vi "Test_Create.vi"(8 "error in (no error)":errorcluster, 11 "TestCase in":refnum<class "StringList_Delegations.lvclass">) -> (0 "error out":errorcluster, 3 "TestCase out":refnum<class "StringList_Delegations.lvclass">)   [LabVIEW 2009, in "StringList_Delegations.lvclass"]
uses:
  StringList_Delegations.lvclass
  Test Doubles/ListImp_RefSpy/ListImp_RefSpy.lvclass
  source/Lists.Interfaces/StringList/StringList.lvclass
  UnitTestComparisons/UnitTestComparisons.lvlib
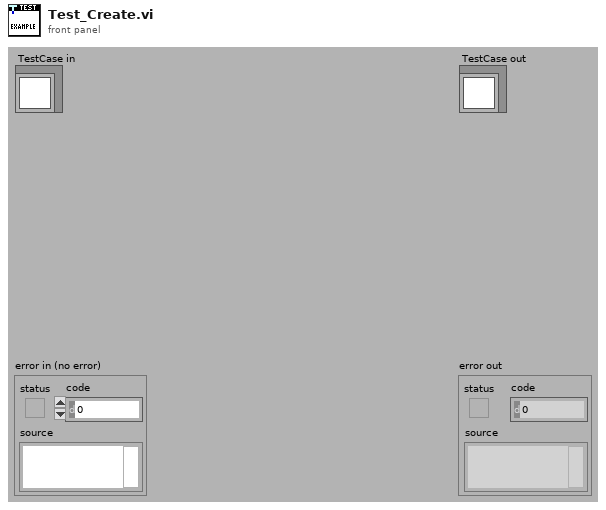
[diagram p1: front panel]
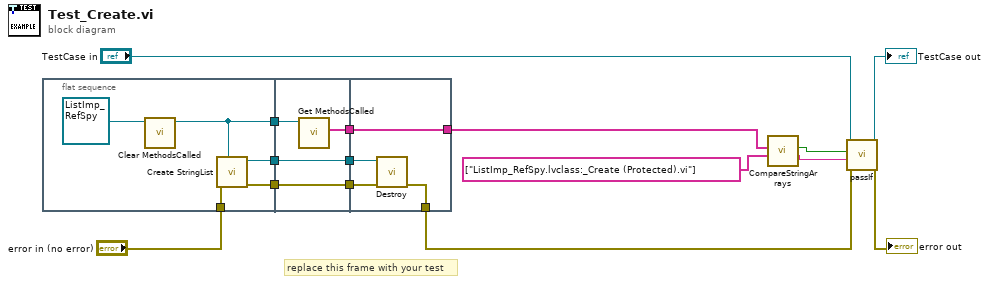
[diagram p0: block diagram]
diagram:
  # "replace this frame with your test"
  n1 = flat-sequence {
    tunnel: [w16] -> w12
    tunnel: [w20] -> w11
    tunnel: [w19] -> w10
    tunnel: "error in (no error)" -> [w18]
    tunnel: w12 -> [w24]
    tunnel: [w23] -> w9
    tunnel: [w22] -> w8
    tunnel: w11 -> [w22]
    tunnel: [w21] -> w7
    tunnel: w10 -> [w21]
    tunnel: [w28] -> w4
    tunnel: w9 -> [w28]
    tunnel: w8 -> [w27]
    tunnel: w7 -> [w26]
    tunnel: [w25] -> w5
    frame #0 {
      n2 = call "Clear MethodsCalled.vi"("MockListImp in"=refnum<class "ListImp_RefSpy.lvclass"> refnum ("MockListImp.lvclass")) -> ("MockListImp out"=w16:refnum<class "ListImp_RefSpy.lvclass">)  [unwired: 9 in, 1 out]
      n3 = call "Create StringList.vi"("List Implementation (Array)"=w16, "error in (no error)"=w18) -> ("error out"=w19:errorcluster, "StringList out"=w20:refnum<class "StringList.lvclass">)  [unwired: 8 in]
    }
    frame #1 {
      n4 = call "Get MethodsCalled.vi"("MockListImp"=w24) -> ("MethodsCalled"=w23:string[])  [unwired: 9 in, 1 out]
    }
    frame #2 {
      n5 = call-dynamic "Destroy.vi"("error in (no error)"=w26, "StringList in"=w27) -> ("error out"=w25:errorcluster)  [unwired: 9 in]
    }
  }
  n6 = call "CompareStringArrays.vi"("Expected Strings"=string[] ["ListImp_RefSpy.lvclass:_Create (Protected).vi"] ("MethodsCalled"), "Actual Strings"=w4) -> ("Message"=w1:string, "Equal?"=w2:bool)  [unwired: 8 in]
  n7 = call-dynamic "passIf.vi"("error in (no error)"=w5, "message (\"\")"=w1, "pass"=w2, "TestCase in"="TestCase in") -> ("error out"=→"error out":errorcluster, "TestCase out"=→"TestCase out":refnum<class "StringList_Delegations.lvclass">)  [unwired: 6 in]
